vi "Servo MSMT WCDMA Configure Measure Step.vi"(8 "error in (no error)":errorcluster, 11 "Servo MSMT in":refnum<class "Servo MSMT.lvclass">) -> (0 "error out":errorcluster, 3 "Servo MSMT out":refnum<class "Servo MSMT.lvclass">)   [LabVIEW 2018, in "Servo MSMT.lvlib" / "Servo MSMT.lvclass"]
uses:
  Servo MSMT.lvclass
  C:/Sequence Automation/Plugins/Measurement Interface.lvlibp/Measurement Interface.lvclass
  Plugins/Measurement Interface.lvlibp/Private Methods/Measurement Name/Read Measurement Name.vi
  Plugins/TestStand API Tools (TSAT).lvlibp/Step Actions/TSAT Step Actions.lvlib
  Plugins/Measurement Interface.lvlibp/Measurement Interface.lvclass
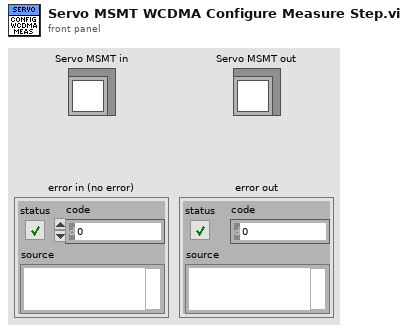
[diagram p1: front panel]
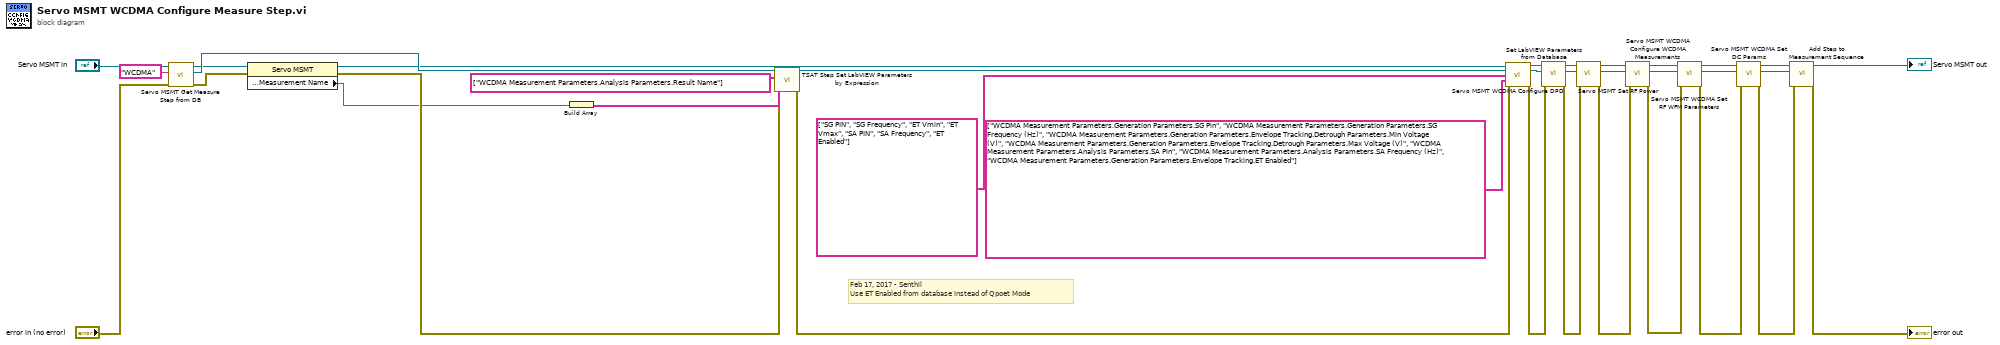
[diagram p0: block diagram]
diagram:
  # "Feb 17, 2017 - Senthil\nUse ET Enabled from database instead of Qpoet Mode"
  n1 = call "Servo MSMT Get Measure Step from DB.vi"("error in (no error)"="error in (no error)", "Standard"="WCDMA", "Servo MSMT in"="Servo MSMT in") -> ("error out"=w13:errorcluster, "Step Out"=w30:refnum<k7>, "Servo MSMT out"=w14:refnum<class "Servo MSMT.lvclass">)  [unwired: 6 in]
  n2 = property class="Servo MSMT"(reference=w14, error in=w13) -> (reference out=w21:refnum<class "Servo MSMT.lvclass">, error out=w32:errorcluster, "Public Methods:Measurement Name"=w16:string)
  n3 = Build Array(w16) -> (w35:string[])
  n4 = call "TSAT Step Set LabVIEW Parameters by Expression.vi"("Error In"=w32, "Value Expressions"=w35, "Parameters to Set"=string[] ["WCDMA Measurement Parameters.Analysis Parameters.Result Name"], "Step In"=w30) -> ("Error Out"=w33:errorcluster, "Step Out"=w31:refnum<k7>)  [unwired: 6 in]
  n5 = call "Set LabVIEW Parameters from Database.vi"("Measurement Interface in"=w21, "Step In"=w31, "Dictionary Keys"=string[] ["SG PIN", "SG Frequency", "ET Vmin", "ET Vmax", "SA PIN", "SA Frequency", "ET Enabled"] ("Database Keys"), "LabVIEW Parameter Mapping"=string[] ["WCDMA Measurement Parameters.Generation Parameters.SG Pin", "WCDMA Measurement Parameters.Generation Parameters.SG Frequency (Hz)", "WCDMA Measurement Parameters.Generation Parameters.Envelope Tracking.Detrough Parameters.Min Voltage (V)", "WCDMA Measurement Parameters.Generation Parameters.Envelope Tracking.Detrough Parameters.Max Voltage (V)", "WCDMA Measurement Parameters.Analysis Parameters.SA Pin", "WCDMA Measurement Parameters.Analysis Parameters.SA Frequency (Hz)", "WCDMA Measurement Parameters.Generation Parameters.Envelope Tracking.ET Enabled"] ("Database Keys"), "error in (no error)"=w33) -> ("Measurement Interface out"=w10:refnum<class "Servo MSMT.lvclass">, "Step Out"=w8:refnum<k7>, "error out"=w15:errorcluster)  [unwired: 8 in]
  n6 = call "Servo MSMT WCDMA Configure DPD.vi"("error in (no error)"=w15, "Step In"=w8, "Servo MSMT in"=w10) -> ("error out"=w11:errorcluster, "Step Out"=w7:refnum<k7>, "Servo MSMT out"=w9:refnum<class "Servo MSMT.lvclass">)  [unwired: 6 in]
  n7 = call-dynamic "Servo MSMT Set RF Power.vi"("error in (no error)"=w11, "Step In"=w7, "Servo MSMT in"=w9) -> ("error out"=w2:errorcluster, "Step Out"=w4:refnum<k7>, "Servo MSMT out"=w6:refnum<class "Servo MSMT.lvclass">)  [unwired: 6 in]
  n8 = call "Servo MSMT WCDMA Configure WCDMA Measurements.vi"("error in (no error)"=w2, "Step In"=w4, "Servo MSMT in"=w6) -> ("error out"=w1:errorcluster, "Step Out"=w3:refnum<k7>, "Servo MSMT out"=w5:refnum<class "Servo MSMT.lvclass">)  [unwired: 6 in]
  n9 = call "Servo MSMT WCDMA Set RF WFM Parameters.vi"("error in (no error)"=w1, "Step In"=w3, "Servo MSMT in"=w5) -> ("error out"=w24:errorcluster, "Step Out"=w18:refnum<k7>, "Servo MSMT out"=w26:refnum<class "Servo MSMT.lvclass">)  [unwired: 6 in]
  n10 = call "Servo MSMT WCDMA Set DC Params.vi"("error in (no error)"=w24, "Step In"=w18, "Servo MSMT in"=w26) -> ("error out"=w25:errorcluster, "Step Out"=w17:refnum<k7>, "Servo MSMT out"=w28:refnum<class "Servo MSMT.lvclass">)  [unwired: 6 in]
  n11 = call "Add Step to Measurement Sequence.vi"("error in (no error)"=w25, "Step to Add"=w17, "Measurement Interface in"=w28) -> ("error out"=→"error out":errorcluster, "Measurement Interface out"=→"Servo MSMT out":refnum<class "Servo MSMT.lvclass">)  [unwired: 7 in]
